vi "Run.vi"(8 "error in (no error)":errorcluster, 11 "fpMgr in":refnum<class "LvProviderShellHelper.lvclass">) -> (0 "error out":errorcluster, 3 "fpMgr out":refnum<class "LvProviderShellHelper.lvclass">)   [LabVIEW 2019, in "LabVIEW-ProviderShell.lvlib" / "LvProviderShellHelper.lvclass"]
uses:
  LvProviderShellHelper.lvclass
  LvProviderShellHelper.lvclass/LvProviderShellHelper.ctl
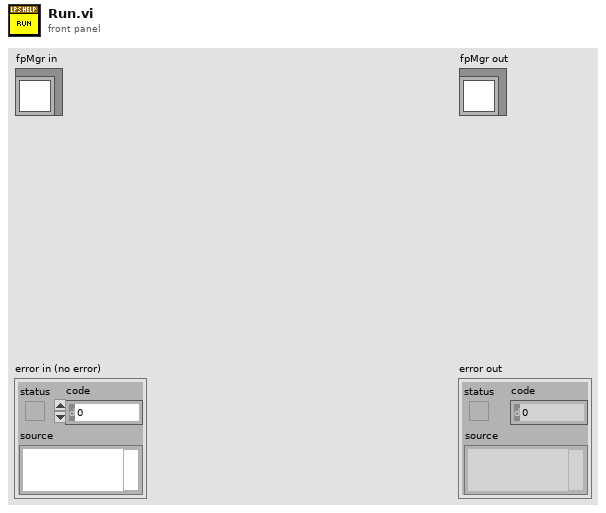
[diagram p1: front panel]
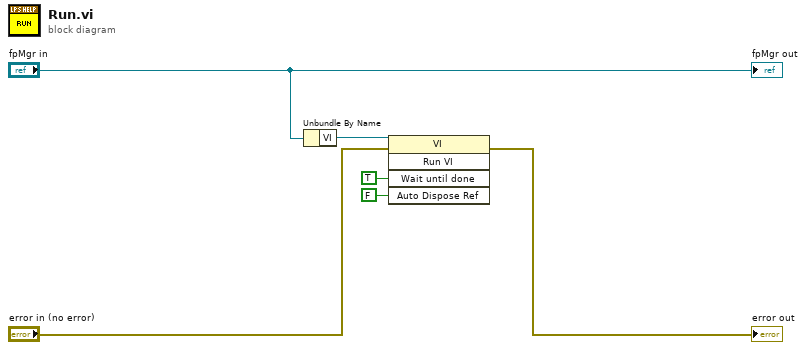
[diagram p0: block diagram]
diagram:
  n1 = Unbundle By Name("fpMgr in") -> ("VI"=w5:refnum<vi>)
  n2 = invoke class="VI" method="Run VI"(reference=w5, error in="error in (no error)", "Wait until done"=TRUE ("Wait Until Done"), "Auto Dispose Ref"=FALSE ("Auto Dispose Reference")) -> (error out=→"error out":errorcluster)  [unwired: 1 in, 4 out]
  "fpMgr out" <- "fpMgr in"
